vi "Dead Band.vi"(9 "Axis In":dbl, 11 "Dead Band":dbl=0.25) -> (2 "Axis Out":dbl)   [LabVIEW 2012]
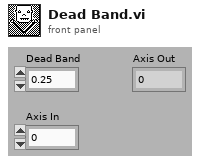
[diagram p1: front panel]
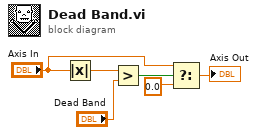
[diagram p0: block diagram]
diagram:
  n1 = Absolute Value(x="Axis In") -> (abs(x)=w2:dbl)
  n2 = Greater?(x=w2, y="Dead Band") -> (0:w1:bool)
  n3 = Select(t="Axis In", s=w1, f=0.0) -> (s? t:f=→"Axis Out":dbl)
